vi "UsrProfiles-Reset scrollbar on first call.vi"(8 "error in (no error)":errorcluster, 11 "ListBox":refnum<vi>) -> (0 "error out":errorcluster)   [LabVIEW 2020]
panel:
  # "Re-entrant VI"
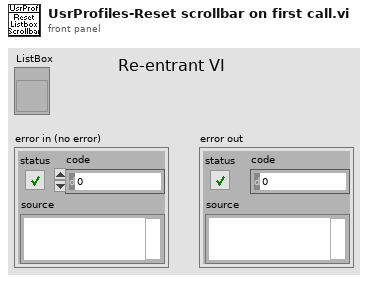
[diagram p1: front panel]
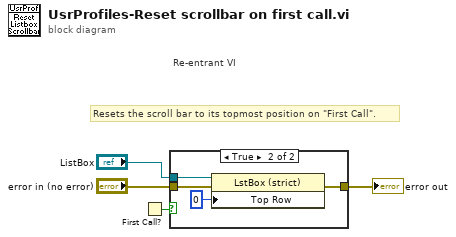
[diagram p0: block diagram]
diagram:
  # "Re-entrant VI"
  # "Resets the scroll bar to its topmost position on \"First Call\"."
  n1 = First Call?() -> (First Call?: T/F=w3:bool)
  n2 = case shown="True" w3 {
    tunnel: "error in (no error)" -> [w5 w9]
    tunnel: [w5 w8] -> w2
    tunnel: "ListBox" -> [_ w7]
    frame False {
    }
    frame True {
      n3 = property class="LstBox (strict)"(reference=w7, error in=w9, "Top Row"=0) -> (error out=w8:errorcluster)  [unwired: 1 out]
    }
  }
  "error out" <- w2
